vi "WaitUIShutDown.vi"   [LabVIEW 2018]
panel:
  # "关闭中...."
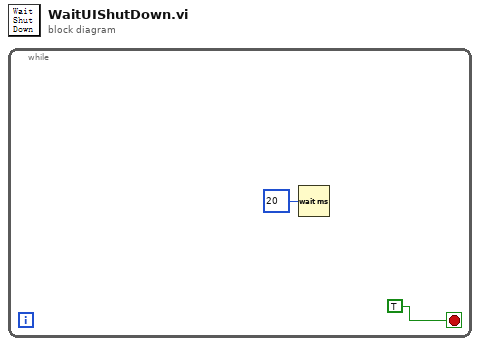
[diagram p0: block diagram]
diagram:
  n1 = while {
    stop <- TRUE stop-if-true
    n2 = Wait (ms)(milliseconds to wait=u32 20 ("等待时间（毫秒）")) -> ()  [unwired: 1 out]
  }
